vi "PID Calculate D.vi"(8 "Change in Time":u32, 9 "Gains":cluster{"P":dbl, "I":dbl, "D":dbl}, 10 "Last Error":dbl, 11 "Error":dbl) -> (3 "Numeric":dbl)   [LabVIEW 2014]
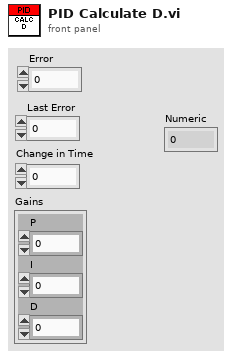
[diagram p1: front panel]
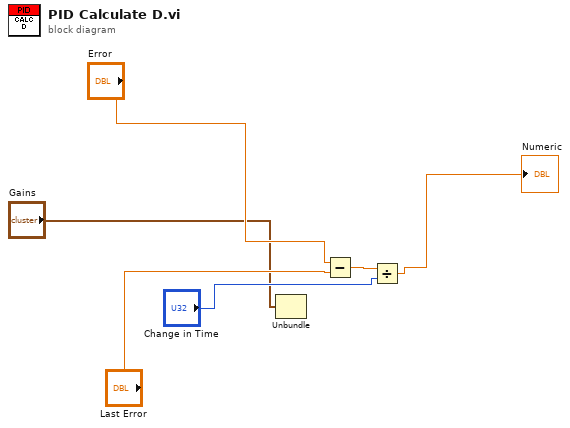
[diagram p0: block diagram]
diagram:
  n1 = Unbundle("Gains") -> ()  [unwired: 3 out]
  n2 = Subtract(x="Error", y="Last Error") -> (x-y=w4:dbl)
  n3 = Divide(x=w4, y="Change in Time") -> (x/y=→"Numeric":dbl)
